vi "VI1.vi"   [LabVIEW 2012]
uses:
  <vilib>/eio/EIONode/EIONode.xnode
  <vilib>/rvi/eio/common/nirviEmuTemplateMethod_errors.vi
  <vilib>/eio/EIOGrowableMethodNode/genericMethod/EIOGrowableMethodNode.xnode
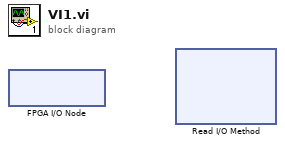
[diagram p0: block diagram]
diagram:
  n1 = xnode "FPGA I/O Node"() -> ()  [unwired: 1 in, 2 out]
  n2 = xnode "Read I/O Method"() -> ()  [unwired: 3 in, 4 out]
